vi "Table Header.vi"(5 "TableHeader out":string[](array[string]), 6 "Row Configuration":T1={"Cell Defaults"={"Background Color"=9868950, "Horizontal Align"=0, "Vertical Align"=1, "Minimum Height"=0.0, "Fixed Height"=0.0, "Padding"={"Left"=2.0, "Top"=2.0, "Right"=2.0, "Bottom"=3.0}}, "Row Borders"={"Left"={"Enabled"=TRUE, "Width"=0.5, "Color"=0}, "Top"={"Enabled"=TRUE, "Width"=0.75, "Color"=0}, "Right"={"Enabled"=TRUE, "Width"=0.5, "Color"=0}, "Bottom"={"Enabled"=TRUE, "Width"=0.75, "Color"=0}, "Middle Vertical"={"Enabled"=TRUE, "Width"=0.5, "Color"=0}}} {"Cell Defaults"."Vertical Align" items=["Bottom", "Middle", "Top"]; "Cell Defaults"."Horizontal Align" items=["Center", "Justified", "JustifiedAll", "Left", "Right"]}, 7 "TableHeader empty?":bool, 8 "Fehler (Eingang, kein Fehler)":errorcluster, 9 "Font":T4={"Font"="Arial", "Size"=10, "Colour"=16777226, "Bold"=TRUE, "Italic"=FALSE, "Underline"=FALSE, "Strikethrough"=FALSE, "Font Encoding"=enum."Cp1252, WinANSI"}, 10 "Table Builder (Eingang)":refnum<class "Table Builder.lvclass">, 11 "Context (Eingang)":refnum<class "Context.lvclass">) -> (0 "Fehler (Ausgang)":errorcluster, 2 "Table Builder (Ausgang)":refnum<class "Table Builder.lvclass">, 3 "Context (Ausgang)":refnum<class "Context.lvclass">)   [LabVIEW 2020, in "PDF Interface.lvlib" / "PDF Interface Helper.lvlib"]
uses:
  <vilib>/Simplicity AI/SAI_PDF_API/Classes/Table Builder/Table Builder.lvclass
  <vilib>/Simplicity AI/SAI_PDF_API/Classes/Context/Context.lvclass
  <vilib>/Simplicity AI/SAI_PDF_API/Classes/Context/Controls/SAI_PDF_Font.ctl
  <vilib>/Simplicity AI/SAI_PDF_API/Classes/Context/Controls/SAI_PDF_Font Encoding.ctl
  <vilib>/Simplicity AI/SAI_PDF_API/Classes/Table Builder/Controls/SAI_PDF_Row Configuration.ctl
  <vilib>/Simplicity AI/SAI_PDF_API/Classes/Table Builder/Controls/SAI_PDF_Default Cell Format.ctl
  <vilib>/Simplicity AI/SAI_PDF_API/Classes/Table Builder/Controls/SAI_PDF_BorderLine.ctl
  PDF Interface Helper.lvlib
panel:
  # "(Cp1252)"
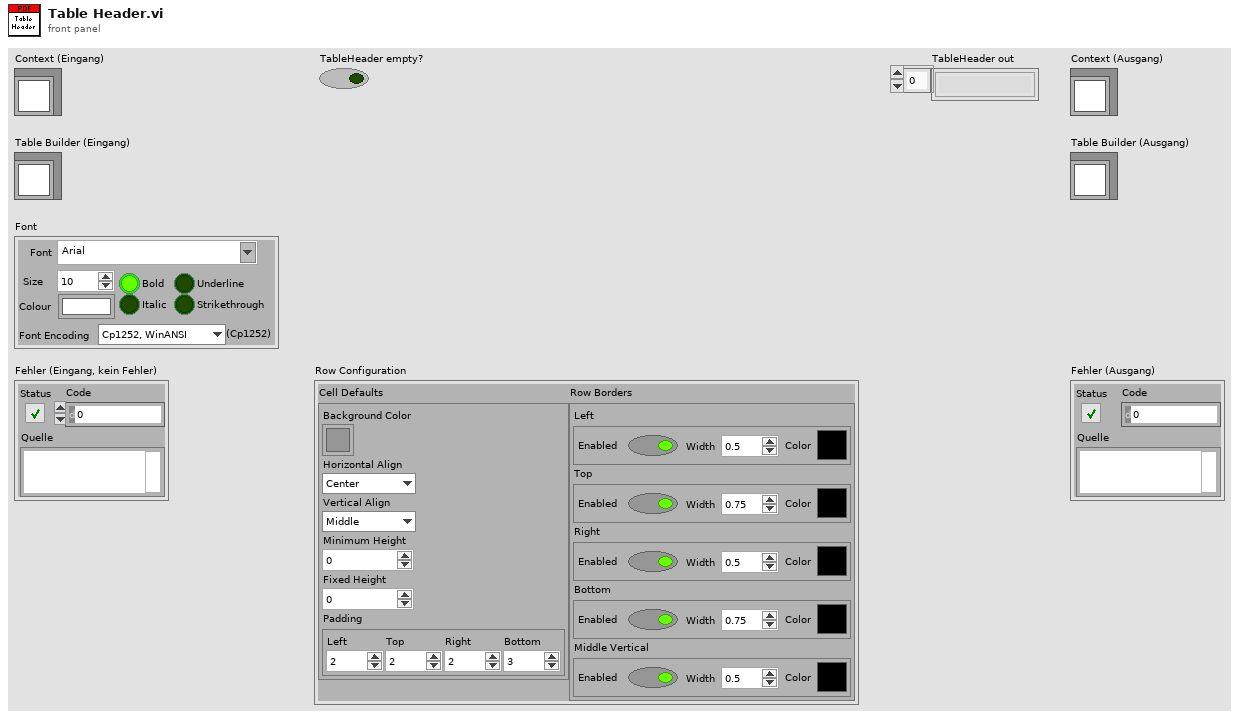
[diagram p1: front panel]
types:
  T1 = typedef "SAI_PDF_Toolkit.lvlib/Table Builder.lvclass/SAI_PDF_Row Configuration.ctl" = cluster{"Cell Defaults":T2, "Row Borders":cluster{"Left":T3, "Top":T3, "Right":T3, "Bottom":T3, "Middle Vertical":T3}}
  T2 = typedef "SAI_PDF_Toolkit.lvlib/Table Builder.lvclass/SAI_PDF_Default Cell Format.ctl" = cluster{"Background Color":u32, "Horizontal Align":i32, "Vertical Align":i32, "Minimum Height":sgl, "Fixed Height":sgl, "Padding":cluster{"Left":sgl, "Top":sgl, "Right":sgl, "Bottom":sgl}}
  T3 = typedef "SAI_PDF_Toolkit.lvlib/Table Builder.lvclass/SAI_PDF_BorderLine.ctl" = cluster{"Enabled":bool, "Width":sgl, "Color":u32}
  T4 = typedef "SAI_PDF_Toolkit.lvlib/Context.lvclass/SAI_PDF_Font.ctl" = cluster{"Font":string, "Size":i32, "Colour":u32, "Bold":bool, "Italic":bool, "Underline":bool, "Strikethrough":bool, "Font Encoding":T5}
  T5 = typedef "SAI_PDF_Toolkit.lvlib/Context.lvclass/SAI_PDF_Font Encoding.ctl" = enum16{"Cp1252, WinANSI", "IdentityH", "IdentityV", "Cp1250", "Cp1257", "MacRoman"}
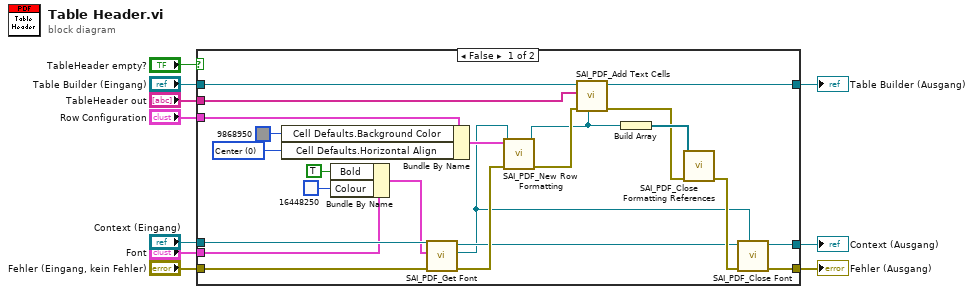
[diagram p0: block diagram]
diagram:
  n1 = case shown="False" "TableHeader empty?" {
    tunnel: "Row Configuration" -> [w33 _]
    tunnel: "Table Builder (Eingang)" -> [w32 w34]
    tunnel: "TableHeader out" -> [w27 _]
    tunnel: "Font" -> [w23 _]
    tunnel: "Context (Eingang)" -> [w30 w36]
    tunnel: [w12 w36] -> w6
    tunnel: "Fehler (Eingang, kein Fehler)" -> [w29 w35]
    tunnel: [w14 w34] -> w9
    tunnel: [w15 w35] -> w10
    frame False {
      w17 = 0 items=["Center", "Justified", "JustifiedAll", "Left", "Right"] ("Horizontal Align")
      n2 = Bundle By Name(cluster=w33, "Cell Defaults.Background Color"=u32 9868950, "Cell Defaults.Horizontal Align"=w17) -> (w19:T1)
      n3 = Bundle By Name(cluster=w23, "Bold"=TRUE, "Colour"=u32 16448250) -> (w22:T4)
      n4 = call <vilib>:"SAI_PDF_Get Font.vi"("error in"=w29, "Font"=w22, "Context In"=w30) -> ("error out"=w28:errorcluster, "Font"=w11:refnum<class "Font.lvclass">, "Context Out"=w13:refnum<class "Context.lvclass">)  [unwired: 6 out]
      n5 = call <vilib>:"SAI_PDF_New Row Formatting.vi"("error in"=w28, "Font In"=w11, "Row Configuration"=w19) -> ("error out"=w31:errorcluster, "Row Formatting"=w26:refnum<class "Formatting.lvclass">)  [unwired: 7 out]
      n6 = call <vilib>:"SAI_PDF_Add Text Cells.vi"("Formatting In"=w26, "error in"=w31, "Cell Text"=w27, "Table Builder In"=w32) -> ("error out"=w24:errorcluster, "Table Builder Out"=w14:refnum<class "Table Builder.lvclass">)  [unwired: 6 out]
      n7 = Build Array(w26) -> (w25:refnum<class "Formatting.lvclass">[])
      n8 = call <vilib>:"SAI_PDF_Close Formatting References.vi"("error in"=w24, "Formatting Refs"=w25) -> ("error out"=w16:errorcluster)  [unwired: 9 out]
      n9 = call <vilib>:"SAI_PDF_Close Font.vi"("Font"=w11, "error in"=w16, "Context In"=w13) -> ("error out"=w15:errorcluster, "Context Out"=w12:refnum<class "Context.lvclass">)  [unwired: 7 out]
    }
    frame True {
    }
  }
  "Fehler (Ausgang)" <- w10
  "Table Builder (Ausgang)" <- w9
  "Context (Ausgang)" <- w6
